vi "GetAlazar_PassData - ATS-SDK.vi"(1 "lines per plane":i32, 5 "File Array":string[](array[string]), 7 "Digitizer Settings":T1={"Digitizer delay (us) "=0.0, "rf points per line"=2048, "lines per plane"=128, "Samp Rate (Hz)"=100000000.0, "Additional dig delay (us)"=0.0, "Voltage Scale"=0.4, "Pre-Looks"=0, "Offset delay (us)"=0.0, "bits A/D"=8, "Avg Num"=1, "DigTimeOut"=5.0, "Rel Dig Delay"=0.0, "Dig Ch"=0, "LeCroyCluster"={"LeCroy Channels"=[TRUE, FALSE, FALSE, FALSE], "LC read pt offset"=0.0, "Sweep Avg"=FALSE}, "Main Digitizer"=enum."NI Digitizer", "Dig Config"=enum."Single channel", "Digitizer ID Cluster"={"Acqiris/Alazar/SP ID"=[], "NI Instr Handles"=[], "LeCroy VISA"="", "GaGe Handle"={"Handle"=0, "Sample size"=0, "Resolution"=0, "Offset"=0, "Channels"=0, "Boards"=0}, "ATS Ref"="ATS9350", "Acqiris Address"=["PCI::INSTR0"], "ADQRef"=refnum, "adq_cu_ptr"=refnum}, "Trigger Settings"={"Trig Source"=1, "Trig Coupling"=0, "Trig Slope"=0, "Level (mV)"=1500.0}, "Bulk Acq"=FALSE, "Bulk Start Indexes"=[], "Data Ref RF"=refnum, "NI ID/Channel"=[], "Total Dig CH"=1, "Xtra Ann Trig delay (us)"=10.0, "Fix Z Delay?"=FALSE, "One Way Transmission?"=FALSE, "Data Ref Log"=refnum} {"Trigger Settings"."Trig Slope" items=["Positive", "Negative"]; "Trigger Settings"."Level (mV)" format="%.2f"; "Trigger Settings"."Trig Coupling" items=["DC 1 MOhm", "AC 1 MOhm", "DC 50 Ohm", "AC 50 Ohm"]; "Trigger Settings"."Trig Source" items=["Chan 1", "External"]; "Rel Dig Delay" format="%.2f"; "DigTimeOut" format="%.2f"; "Avg Num" min=1; "Offset delay (us)" format="%.2f"; "Additional dig delay (us)" format="%.2f"; "Digitizer delay (us)" format="%.2f"}, 9 "AlazarCluster":T5, 11 "error in":errorcluster, 13 "Reverse?":bool) -> (3 "VGain (dB)":dbl, 6 "Gain Array":T7(array[cluster]), 8 "Array out":i16[][][](array[numeric]), 14 "Raw VGain (scale)":dbl, 15 "error out":errorcluster)   [LabVIEW 2022 SP3]
uses:
  -DigitizerRoutines/DigitizerSettings.ctl
  -DigitizerRoutines/Digitizer.ctl
  -DigitizerRoutines/DigConfig.ctl
  -DigitizerRoutines/DigitizerID.ctl
  C:/Windows/System32/ADQAPI_dotNet_helper.dll
  -ScanSystem/DataHandling/ReverseData.vi
panel:
  out "Voltage Scale":T6
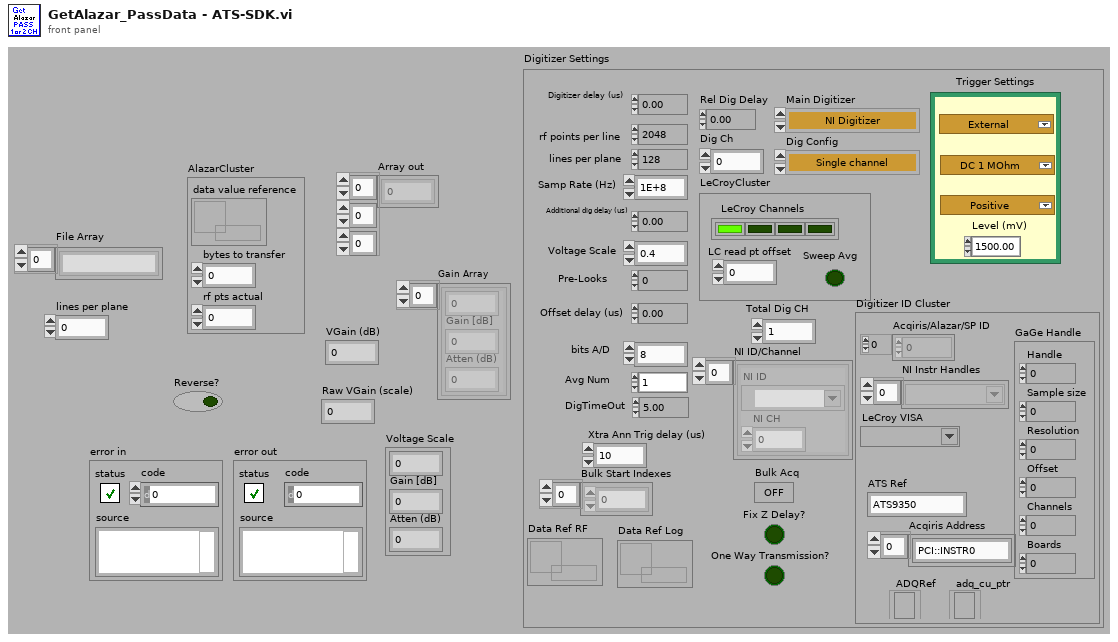
[diagram p1: front panel]
types:
  T1 = typedef "DigitizerSettings.ctl" = cluster{"Digitizer delay (us) ":dbl, "rf points per line":i32, "lines per plane":i32, "Samp Rate (Hz)":dbl, "Additional dig delay (us)":dbl, "Voltage Scale":dbl, "Pre-Looks":i32, "Offset delay (us)":dbl, "bits A/D":i8, "Avg Num":i32, "DigTimeOut":sgl, "Rel Dig Delay":sgl, "Dig Ch":i32, "LeCroyCluster":cluster{"LeCroy Channels":bool[], "LC read pt offset":dbl, "Sweep Avg":bool}, "Main Digitizer":T2, "Dig Config":T3, "Digitizer ID Cluster":T4, "Trigger Settings":cluster{"Trig Source":u16, "Trig Coupling":u16, "Trig Slope":u16, "Level (mV)":dbl}, "Bulk Acq":bool, "Bulk Start Indexes":i32[], "Data Ref RF":refnum<data-value>, "NI ID/Channel":cluster{"NI ID":refnum<k15>, "NI CH":i32}[], "Total Dig CH":i32, "Xtra Ann Trig delay (us)":dbl, "Fix Z Delay?":bool, "One Way Transmission?":bool, "Data Ref Log":refnum<data-value>}
  T2 = typedef "Digitizer.ctl" = enum16{"Acqiris Digitizer", "NI Digitizer", "LeCroy", "GaGe", "AlazarTech", "No Digitizer", "Teledyne"}
  T3 = typedef "DigConfig.ctl" = enum16{"Single channel", "2 Chans w/ 2 Acqiris", "2 Chans w/ 1 Acqiris", "5-CH Pulser New", "5-CH pulser w/ ann array", "5-pass style ann array", "Empty"}
  T4 = typedef "DigitizerID.ctl" = cluster{"Acqiris/Alazar/SP ID":u32[], "NI Instr Handles":refnum<k15>[], "LeCroy VISA":refnum<visa-resource-name>, "GaGe Handle":cluster{"Handle":u32, "Sample size":u32, "Resolution":i32, "Offset":i32, "Channels":u32, "Boards":u32}, "ATS Ref":string, "Acqiris Address":string[], "ADQRef":refnum<k24>, "adq_cu_ptr":refnum<k24>}
  T5 = cluster{"data value reference":refnum<data-value>, "bytes to transfer":u32, "rf pts actual":u32}
  T6 = cluster{sgl, "Gain [dB]  ":sgl, "Atten (dB)":sgl}
  T7 = cluster{sgl, "Gain [dB]  ":sgl, "Atten (dB)":sgl}[]
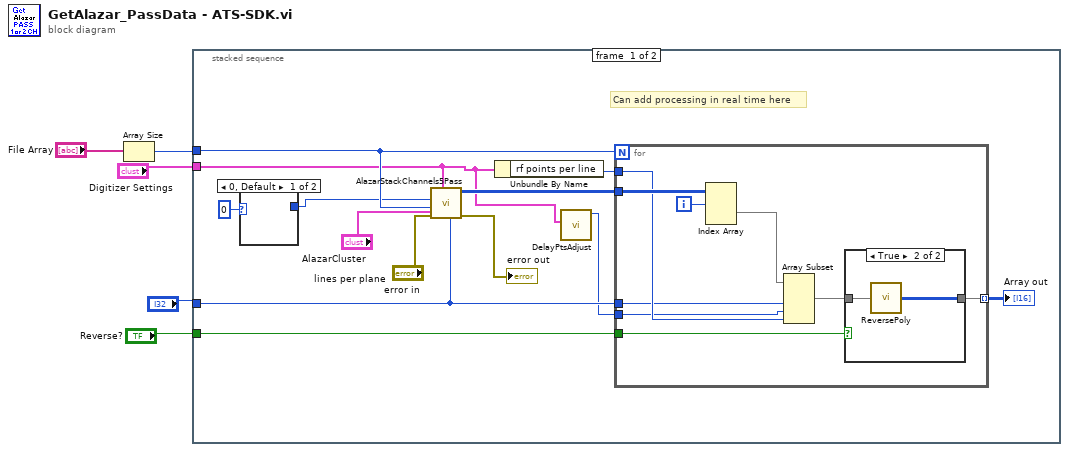
[diagram p0: block diagram]
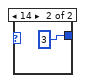
[diagram p2: hidden frame]
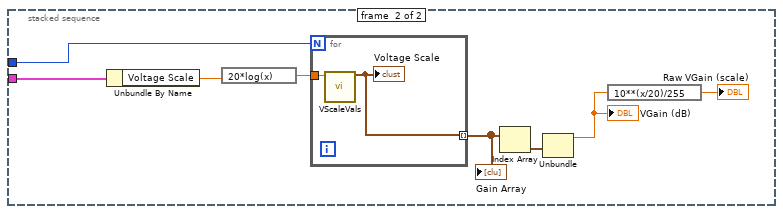
[diagram p4: hidden frame]
diagram:
  n1 = Array Size(array="File Array") -> (size(s)=w5:i32)
  n2 = stacked-sequence {
    tunnel: "lines per plane" -> [w11 _]
    tunnel: "Reverse?" -> [w18 _]
    tunnel: w5 -> [w10 w38]
    tunnel: "Digitizer Settings" -> [w7 w33]
    frame #0 {
      # "Can add processing in real time here"
      n3 = case shown="0, Default" i8 0 ("bits A/D") {
        tunnel: [_ u16 3 ("Extra Shift")] -> w8
        frame 0, Default {
        }
        frame 14 {
        }
      }
      n4 = call "AlazarStackChannels5Pass.vi"("lines per plane"=w11, "AlazarCluster"="AlazarCluster", "Digitizer Settings"=w7, "error in"="error in", "Channels"=w10, "Extra Shift"=w8) -> ("error out"=→"error out":errorcluster, "ChStackDataOut"=w15:i16[][][])  [unwired: 2 in, 2 out]
      n5 = Unbundle By Name(w7) -> ("rf points per line"=w16:i32)
      n6 = call "DelayPtsAdjust.vi"("Digitizer Settings"=w7) -> ("PostDelayCorrection"=w6:u32)  [unwired: 9 in, 1 out]
      n7 = for {
        N: w10 -> [_]
        tunnel: w15 -> [w28]
        tunnel: w16 -> [w27]
        tunnel: w11 -> [w26]
        tunnel: w18 -> [w25]
        tunnel: [w21] -> w17 mode=indexing
        tunnel: w6 -> [w20]
        i -> [w22]
        n8 = Index Array(array=w28, index (dim 0)=w22) -> (element=w23:i16[][])  [unwired: 2 in]
        n9 = Array Subset(array=w23, length (row)=w26, index (col)=w20, length (col)=w27) -> (w24:i16[][])  [unwired: 1 in]
        n10 = case shown="True" w25 {
          tunnel: [w29 w31] -> w21
          tunnel: w24 -> [w29 w30]
          frame False {
          }
          frame True {
            n11 = call-poly "ReversePoly.vi"("Array in"=w30) -> ("Array out"=w31:i16[][])
          }
        }
      }
      "Array out" <- w17
    }
    frame #1 {
      n12 = Unbundle By Name(w33) -> ("Voltage Scale"=w32:dbl)
      n13 = expression code="20*log(x)"(w32) -> (w39:dbl)
      n14 = for {
        N: w38 -> [_]
        tunnel: [w40] -> w34 mode=indexing
        tunnel: w39 -> [w41]
        n15 = call "VScaleVals.vi"("Full Scale"=w41) -> ("Voltage Scale"=w40:T6)  [unwired: 8 in, 2 out]
        "Voltage Scale" <- w40
      }
      "Gain Array" <- w34
      n16 = Index Array(array=w34) -> (element=w37:T6)  [unwired: 1 in]
      n17 = Unbundle(w37) -> (w36:sgl)  [unwired: 2 out]
      "VGain (dB)" <- w36
      n18 = expression code="10**(x/20)/255"(w36) -> (→"Raw VGain (scale)":sgl)
    }
  }
